vi "asap_stage_calibration.vi"() -> ()   [LabVIEW 2013]
uses:
  <vilib>/Platform/TimedLoop/XDataNode/XDataNode.xnode
  <vilib>/Platform/TimedLoop/XDataNode/nitl_modes.ctl
  <vilib>/Platform/TimedLoop/XDataNode/XDNodeRunTimeDep.lvlib
  <vilib>/Platform/TimedLoop/XDataNode/wakeup.ctl
  <vilib>/Platform/TimedLoop/XDataNode/timing_clust.ctl
  initialization/micron_globals.vi
  <vilib>/Analysis/Matrix/Datatypes/RealMatrix.ctl
  <vilib>/Analysis/Matrix/NI_Matrix.lvlib
  point_selector.ctl
panel:
  in  "Point selector":T1={"Pose mode"=enum."Handle", "Light number"=0} {"Light number" min=0 max=5}
  in  "Pessimize":bool
  in  "Zero Rx":bool
  in  "Home pose offset":dbl[](array[numeric])=[0.0, 0.0, 0.0, 0.0, 0.0, 0.0] format="%#.3f"
  in  "End transform offset":dbl[](array[numeric])=[0.0, 0.0, 0.0, 0.0, 0.0, 0.0] format="%#.3f"
  in  "Update axes":bool
  out "Axis offsets":dbl[](array[numeric])=[0.09384767289236115, -1.0269022597345072, 2.2800407915457908] format="%#.3g"
  in  "LED enable":bool[](array[boolean])=[TRUE, TRUE, TRUE, TRUE, TRUE, TRUE]
  out "Axis scale errors (percent)":sgl[](array[numeric]) format="%#.2f"
  out "End transform string":string
  in  "End transform\ncoordinates":T2(ring)=enum."ASAP"
  in  "Go home":bool
  in  "Clear":bool
  in  "Set home":bool
  out "End transform (stage)":dbl[](array[numeric])=[0.25469575119784055, -16.45995133588347, 3.732397870471535, 0.0, 0.0, 0.0] format="%#.3f"
  in  "Range (degrees)":dbl=40.0 caption="(degrees)"
  in  "Range (mm)":dbl=50.0 caption="(mm)"
  out "Goal pose ASAP string":string
  out "Probe rotation (stage)":T3 format="%#_3f"
  out "Light rotation string":string
  out "Light pose string":string
  out "Probe pose (ASAP)":T3 format="%#_3f"
  out "State orientation string":string
  out "ASAP origin (Base)":dbl[](array[numeric])=[0.0, 0.0, 0.0, 0.0, 0.0, -30.0] format="%#_3p"
  out "Home pose (base)":dbl[](array[numeric])=[0.25469575119784055, -16.45995133588347, 3.732397870471535, 0.0, 0.0, 0.0] format="%#.3f"
  out "Goal pose (stage)":dbl[](array[numeric])=[0.0, 0.0, 0.0, 0.0, 0.0, -30.0] format="%#_3p"
  in  "Go to":bool
  in  "Probe goal pose (ASAP)":dbl[](array[numeric])=[0.0, 0.0, 0.0, 0.0, 0.0, 180.0]
  in  "Update pivot":bool
  out "Off axis":dbl[](array[numeric]) format="%#_3p"
  in  "Pivot point (mm)":dbl[](array[numeric])=[0.09384767289236115, -1.0269022597345072, 2.2800407915457908] format="%#.3g"
  out "Center offsets  (um)":dbl[][](array[numeric]) format="%#_3p"
  in  "Axes":i32[](array[numeric])=[0, 1, 2]
  in  "Find center":bool
  in  "stop":bool
  in  "Find pose":bool
  out "Axis angle errors (radians)":dbl[](array[numeric]) format="%#_3p"
  out "Base orientation (ASAP)":T3 format="%#_3f"
  # "Range limits"
  # "XY"
  # "XZ"
  # "YZ"
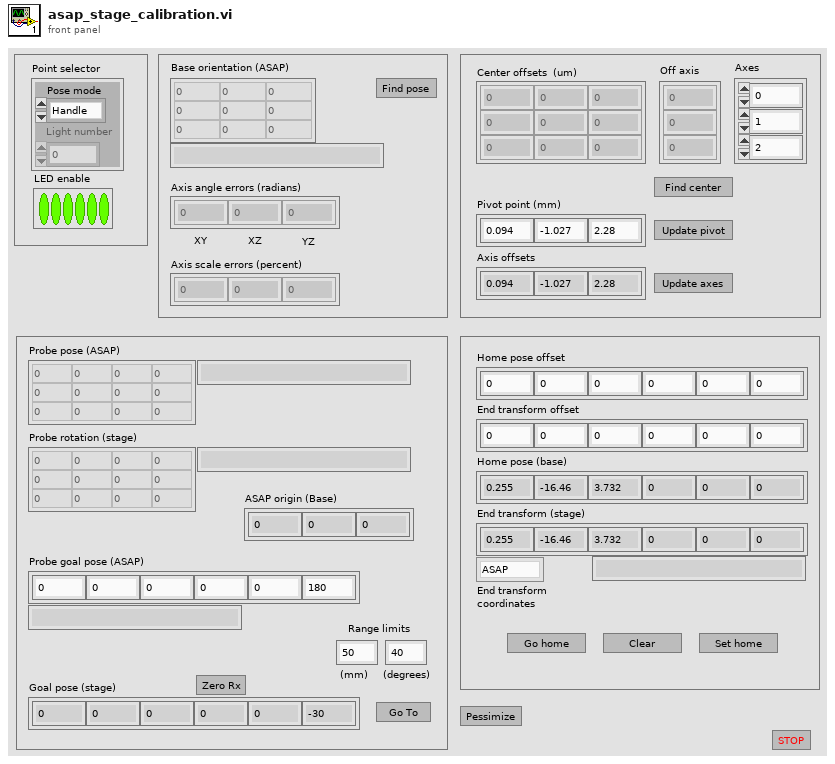
[diagram p1: front panel]
types:
  T1 = typedef "point_selector.ctl" = cluster{"Pose mode":enum16{"Light", "Handle", "Output"}, "Light number":i32}
  T2 = enum16{"Pivot", "Probe", "ASAP", "Sensor 0", "Sensor 1"}
  T3 = typedef "NI_Matrix.lvlib/RealMatrix.ctl" = dbl[][]
  T4 = typedef "ui_override_opts.ctl" = cluster{"Triggering":bool, "Parameters":bool, "Stimulus":bool, "Calibration":bool, "Modes":bool}
  T5 = enum8{"Enabled", "Disabled", "Disabled and Grayed Out"}
  T6 = typedef "XDNodeRunTimeDep.lvlib/timing_clust.ctl" = cluster{"Expected End [f-1]":u64, "Actual End [f-1]":u64, "Finished Late? [f-1]":bool, "Expected End [i-1]":u64, "Actual End [i-1]":u64, "Finished Late? [i-1]":bool, "Expected Start [i]":u64, "Actual Start [i]":u64, "Expected Start [f]":u64, "Actual Start [f]":u64, "Source Name":string, "Structure Name":string, "Period":i64, "Deadline":i64, "Offset":i64, "Start":i64, "Priority":i32, "Timeout":i32, "Mode":T7, "Wakeup Reason":T8, "Error":errorcluster, "Source Type":string, "Secondary Source Type":string, "Global End Time":u64, "Global Start Time":u64, "Frame Duration":u64, "Iteration Duration":u64, "Assigned CPU":i32, "I/O Scan Engine Mode":u32}
  T7 = typedef "XDNodeRunTimeDep.lvlib/nitl_modes.ctl" = enum32{"No Change", "Process missed periods, maintain original phase", "Discard missed periods, maintain original phase", "Process missed periods, ignore original phase", "Discard missed periods, ignore original phase"}
  T8 = typedef "XDNodeRunTimeDep.lvlib/wakeup.ctl" = enum32{"Normal", "Aborted", "Asynchronous wakeup", "Timing source error", "Timed loop error", "Timeout"}
  T9 = typedef "motion_status.ctl" = cluster{"Axis names":string[], "Axis positions":dbl[], "Pose":dbl[], "Timestamp":u32, "Ready":bool, "Stopped":bool}
  T10 = typedef "micron_config.ctl" = cluster{"rt fifo":refnum<k33>, "Analog output task":refnum<k21>, "Analog output task 2":refnum<k21>, "Stimulus AO task":refnum<k21>, "Low-rate AIN task":refnum<k21>, "Pedal out task":refnum<k21>, "Pedal in task":refnum<k21>, "Loop timing source":string, "Relay out task":refnum<k21>, "Send UDP Conn":refnum<k16>, "Recv UDP Conn":refnum<k16>, "Host Addr":dbl, "I2C interface":T11, "trace_start notifier":refnum<notifier>, "trace_done notifier":refnum<notifier>, "ASAP FIFO":refnum<k33>}
  T11 = typedef "i2c_interface.ctl" = cluster{"FPGA VI Reference":T12}
  T12 = typedef "fpga_reference.ctl" = refnum<k20>
  T13 = enum32{"Bad", "Idle", "Run top level", "Running"}
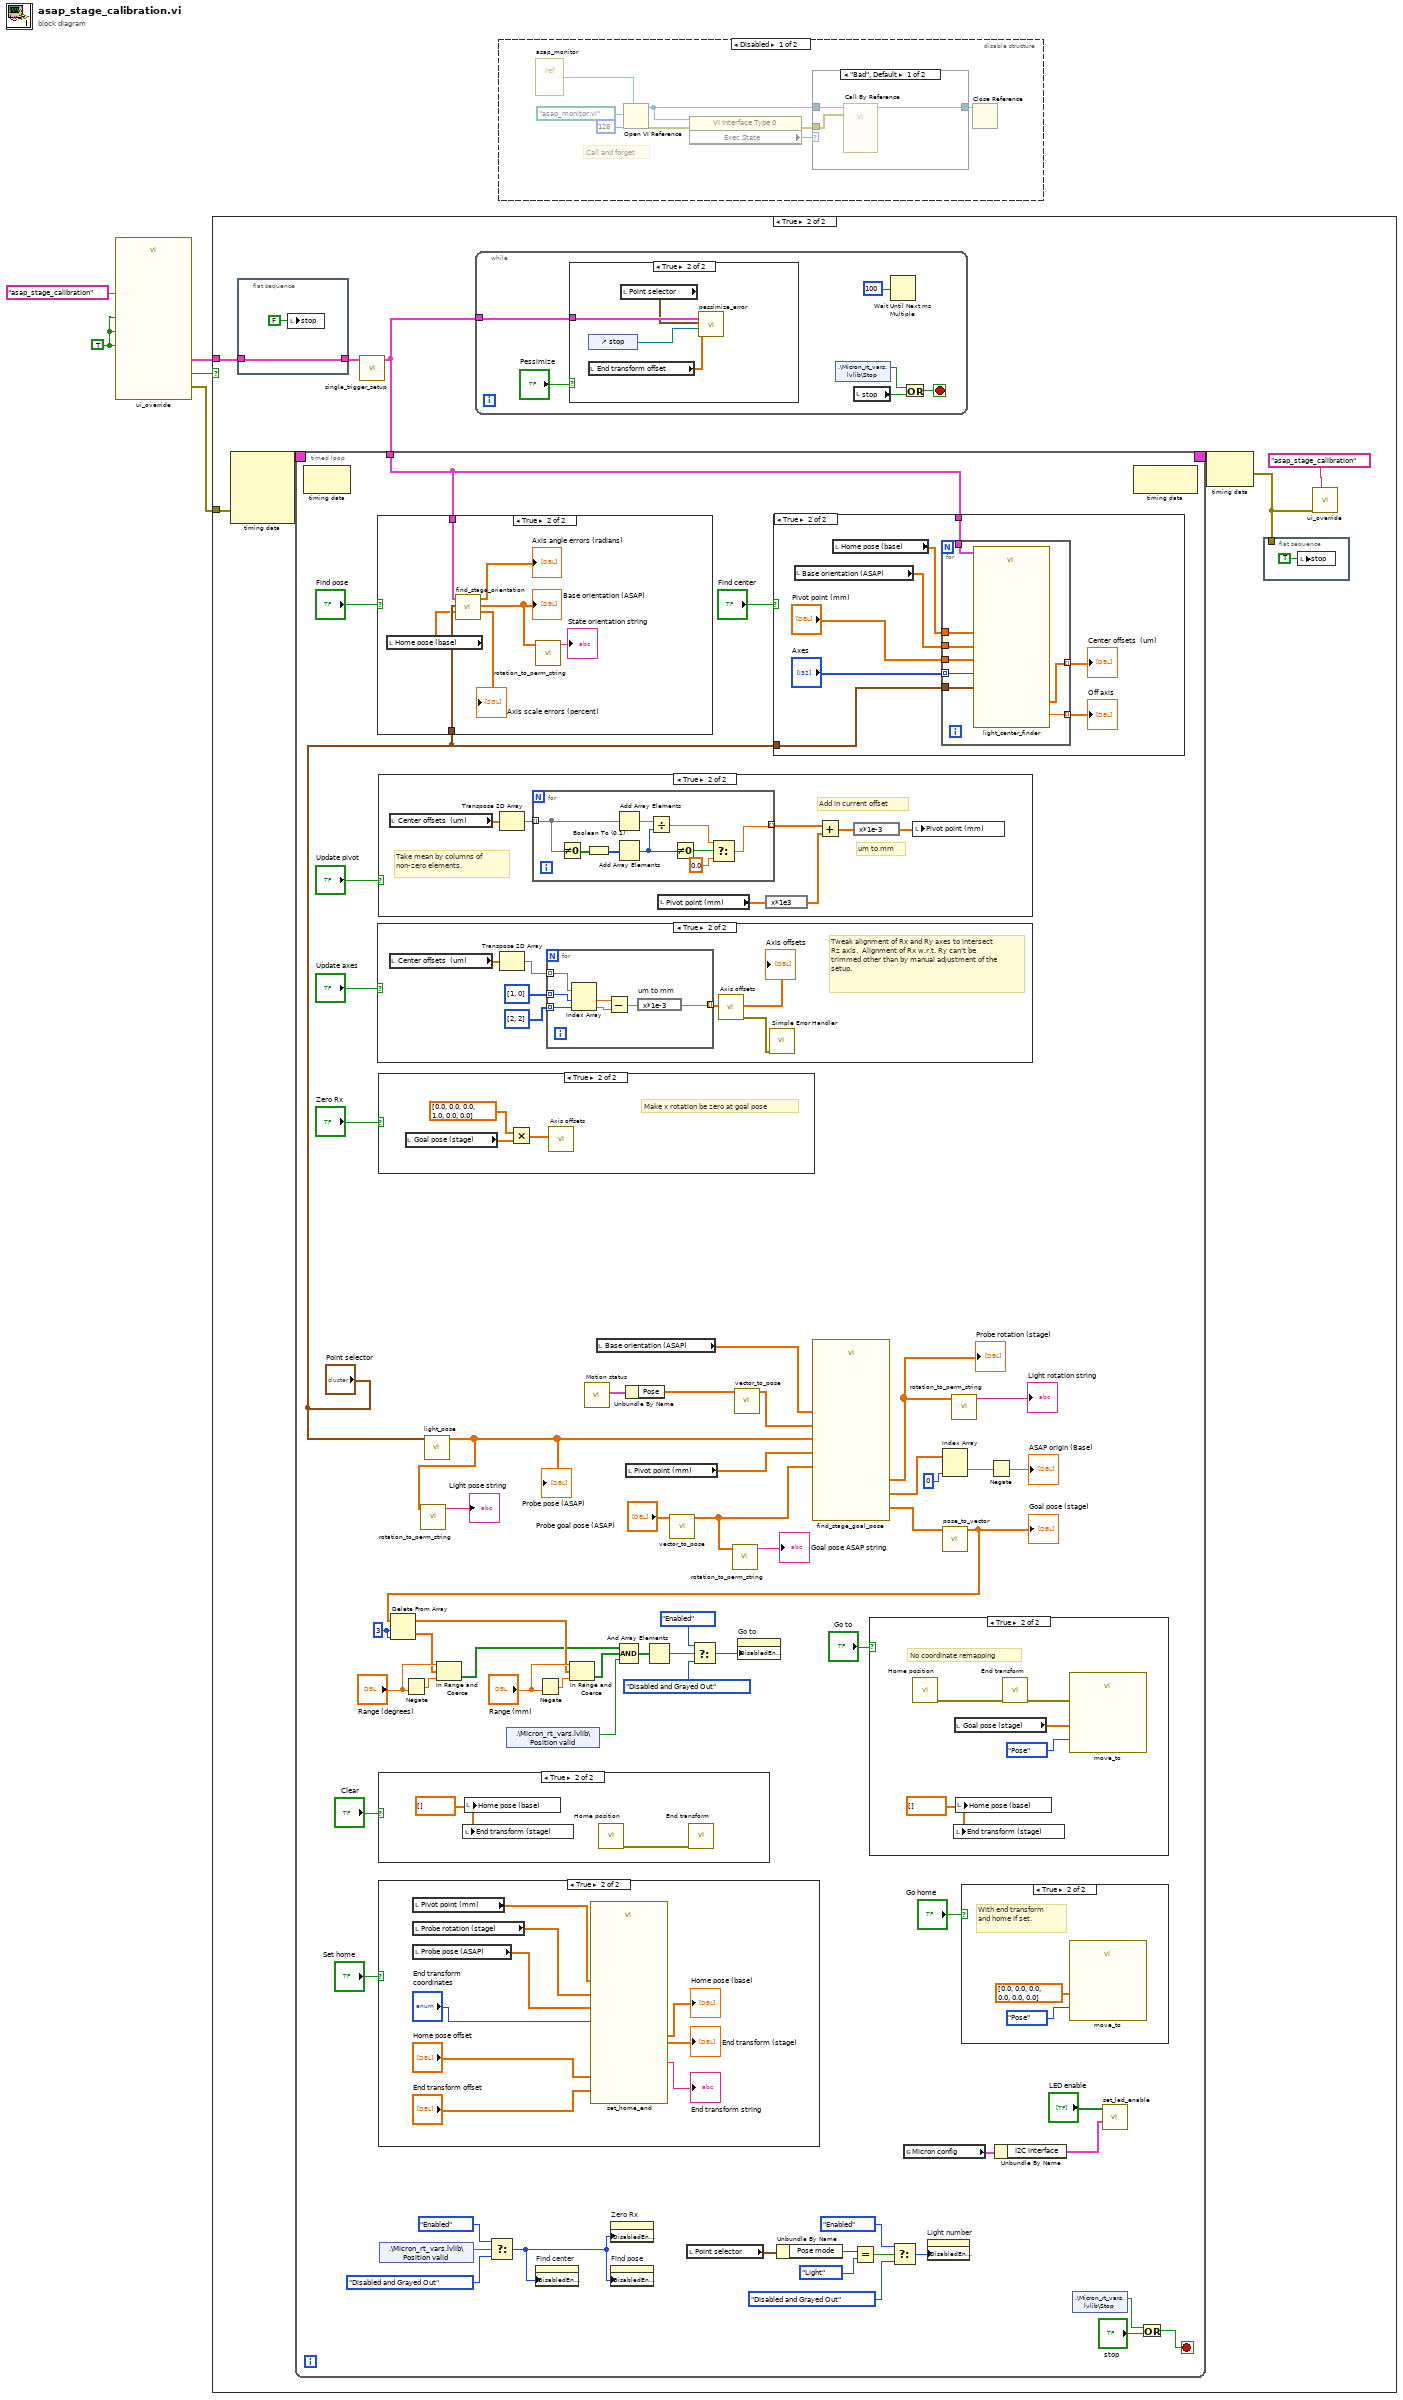
[diagram p0: block diagram]
diagram:
  w3 = TRUE ("Triggering")
  n1 = call "ui_override.vi"("Triggering"=w3, "VI name"="asap_stage_calibration", "Stimulus"=w3, "All or nothing"=w3) -> ("Override"=w2:T4, "Got all"=w5:bool, "error out"=w1:errorcluster)  [unwired: 9 in]
  n2 = case shown="True" w5 {
    tunnel: w1 -> [_ w11]
    tunnel: w2 -> [_ w8]
    frame False {
    }
    frame True {
      n3 = node-c288(w11) -> (w13:T6)  [unwired: 3 in]
      n4 = flat-sequence {
        tunnel: w8 -> [w16]
        tunnel: [w16] -> w9
        frame #0 {
          n5 = local write "stop"(FALSE ("stop")) -> ()
        }
      }
      n6 = call "single_trigger_setup.vi"("Override in"=w9) -> ("Override out"=w7:T4)  [unwired: 10 in]
      n7 = timed-loop {
        timing: w13 -> [_]
        timing-out: [_] -> w12
        tunnel: w7 -> [w83]
        stop <- w84 stop-if-true
        w62 = 3 ("length")
        n8 = node-c288() -> ()  [unwired: 1 in, 1 out]
        n9 = case shown="True" "Find pose" {
          tunnel: w83 -> [_ w161]
          tunnel: "Point selector" -> [_ w159]
          frame False {
          }
          frame True {
            n10 = local read "Home pose (base)"() -> (w158:dbl[])
            n11 = call "find_stage_orientation.vi"("Home pose"=w158, "Point selector"=w159, "Override"=w161) -> ("Axis scale errors (percent)"=→"Axis scale errors (percent)":sgl[], "Stage pose (rotation only)"=w156:T3, "Axis errors (radians)"=→"Axis angle errors (radians)":dbl[])  [unwired: 6 in]
            "Base orientation (ASAP)" <- w156
            n12 = call "rotation_to_perm_string.vi"("Rotation matrix (T)"=w156) -> ("Axis permutation and residue"=→"State orientation string":string)  [unwired: 10 in]
          }
        }
        n13 = case shown="True" "Update axes" {
          frame False {
          }
          frame True {
            # "Tweak alignment of Rx and Ry axes to intersect Rz axis.  Alignment of Rx w.r.t. Ry can't be trimmed other than by manual adjustment of the setup."
            n14 = local read "Center offsets  (um)"() -> (w96:dbl[][])
            n15 = Transpose 2D Array(2D array=w96) -> (transposed array=w95:dbl[][])
            n16 = for {
              tunnel: w95 -> [w102] mode=indexing
              tunnel: i32[] [1, 0] -> [w104] mode=indexing
              tunnel: i32[] [2, 2] -> [w103] mode=indexing
              tunnel: [w98] -> w92 mode=indexing
              n17 = Index Array(array=w102, index #1=w104, index #2=w103) -> (element #1=w101:dbl, element #2=w100:dbl)
              n18 = Subtract(x=w101, y=w100) -> (x-y=w99:dbl)
              n19 = expression code="x*1e-3" "um to mm"(w99) -> (w98:dbl)
            }
            n20 = call "Axis offsets.vi"("Axis offsets increment"=w92) -> ("error out"=w91:errorcluster, "Axis offsets"=→"Axis offsets":dbl[])  [unwired: 9 in]
            n21 = call <vilib>:"Simple Error Handler.vi"("error in (no error)"=w91) -> ()  [unwired: 4 in, 5 out]
          }
        }
        n22 = case shown="True" "Update pivot" {
          frame False {
          }
          frame True {
            # "Add in current offset"
            # "um to mm"
            # "Take mean by columns of non-zero elements."
            n23 = local read "Center offsets  (um)"() -> (w129:dbl[][])
            n24 = Transpose 2D Array(2D array=w129) -> (transposed array=w128:dbl[][])
            n25 = for {
              tunnel: w128 -> [w136] mode=indexing
              tunnel: [w131] -> w126 mode=indexing
              n26 = Not Equal To 0?(x=w136) -> (x != 0?=w138:bool[])
              n27 = Boolean To (0,1)(Boolean=w138) -> (0, 1=w137:i16[])
              n28 = Add Array Elements(numeric array=w136) -> (sum=w135:dbl)
              n29 = Add Array Elements(numeric array=w137) -> (sum=w134:i16)
              n30 = Divide(x=w135, y=w134) -> (x/y=w132:dbl)
              n31 = Not Equal To 0?(x=w134) -> (x != 0?=w133:bool)
              n32 = Select(t=w132, s=w133, f=0.0) -> (s? t:f=w131:dbl)
            }
            n33 = local read "Pivot point (mm)"() -> (w124:dbl[])
            n34 = expression code="x*1e3"(w124) -> (w123:dbl[])
            n35 = Add(x=w126, y=w123) -> (x+y=w125:dbl[])
            n36 = expression code="x*1e-3"(w125) -> (w127:dbl[])
            n37 = local write "Pivot point (mm)"(w127) -> ()
          }
        }
        n38 = case shown="True" "Zero Rx" {
          frame False {
          }
          frame True {
            # "Make x rotation be zero at goal pose"
            n39 = local read "Goal pose (stage)"() -> (w90:dbl[])
            n40 = Multiply(x=dbl[] [0.0, 0.0, 0.0, 1.0, 0.0, 0.0] ("Goal pose (stage)"), y=w90) -> (x*y=w88:dbl[])
            n41 = call "Axis offsets.vi"("Axis offsets increment"=w88) -> ()  [unwired: 9 in, 2 out]
          }
        }
        n42 = case shown="True" "Clear" {
          frame False {
          }
          frame True {
            w107 = dbl[] [] ("Home position")
            n43 = local write "End transform (stage)"(w107) -> ()
            n44 = local write "Home pose (base)"(w107) -> ()
            n45 = call "Home position.vi"() -> ("error out"=w108:errorcluster)  [unwired: 11 in]
            n46 = call "End transform.vi"("error in"=w108) -> ()  [unwired: 10 in, 1 out]
          }
        }
        n47 = case shown="True" "Set home" {
          frame False {
          }
          frame True {
            n48 = local read "Pivot point (mm)"() -> (w116:dbl[])
            n49 = local read "Probe rotation (stage)"() -> (w115:T3)
            n50 = local read "Probe pose (ASAP)"() -> (w112:T3)
            n51 = call "set_home_end.vi"("End transform offset"="End transform offset", "End transform coordinates"="End transform\ncoordinates", "Home pose offset"="Home pose offset", "Probe pose (ASAP)"=w112, "Probe rotation (stage)"=w115, "Pivot point (mm)"=w116) -> ("End transform string"=→"End transform string":string, "End transform"=→"End transform (stage)":dbl[], "Home pose"=→"Home pose (base)":dbl[])  [unwired: 3 in]
          }
        }
        n52 = shared-variable ".\\Micron_rt_vars.lvlib\\Position valid"() -> (w40:bool)  [unwired: 1 in, 1 out]
        n53 = Negate(x="Range (degrees)") -> (-x=w59:dbl)
        n54 = call "light_pose.vi"("Point selector"="Point selector") -> ("Light pose (ASAP coordinates)"=w66:T3)  [unwired: 10 in]
        "Probe pose (ASAP)" <- w66
        n55 = call "rotation_to_perm_string.vi"("Rotation matrix (T)"=w66) -> ("Axis permutation and residue"=→"Light pose string":string)  [unwired: 10 in]
        n56 = Select(t=T5."Enabled" ("Disabled"), s=w40, f=T5."Disabled and Grayed Out" ("Disabled")) -> (s? t:f=w35:T5)
        n57 = shared-variable ".\\Micron_rt_vars.lvlib\\Position valid"() -> (w37:bool)  [unwired: 1 in, 1 out]
        n58 = property on="Find center" class="Bool"("DisabledEnum"=w35) -> ()  [unwired: 2 in, 2 out]
        n59 = Negate(x="Range (mm)") -> (-x=w61:dbl)
        n60 = call "Motion status.vi"() -> ("Motion status"=w79:T9)  [unwired: 6 in, 5 out]
        n61 = local read "Base orientation (ASAP)"() -> (w70:T3)
        n62 = property on="Zero Rx" class="Bool"("DisabledEnum"=w35) -> ()  [unwired: 2 in, 2 out]
        n63 = property on="Find pose" class="Bool"("DisabledEnum"=w35) -> ()  [unwired: 2 in, 2 out]
        n64 = Unbundle By Name(w79) -> ("Pose"=w76:dbl[])
        n65 = local read "Pivot point (mm)"() -> (w77:dbl[])
        n66 = call "vector_to_pose.vi"("Pose vector"="Probe goal pose (ASAP)") -> ("Pose"=w65:T3)  [unwired: 10 in]
        n67 = local read "Point selector"() -> (w29:T1)
        n68 = call "rotation_to_perm_string.vi"("Rotation matrix (T)"=w65) -> ("Axis permutation and residue"=→"Goal pose ASAP string":string)  [unwired: 10 in]
        n69 = call "vector_to_pose.vi"("Pose vector"=w76) -> ("Pose"=w71:T3)  [unwired: 10 in]
        n70 = case shown="True" "Find center" {
          tunnel: w83 -> [_ w146]
          tunnel: "Point selector" -> [_ w145]
          frame False {
          }
          frame True {
            n71 = local read "Base orientation (ASAP)"() -> (w142:T3)
            n72 = local read "Home pose (base)"() -> (w140:dbl[])
            n73 = for {
              tunnel: w146 -> [w154]
              tunnel: w145 -> [w153]
              tunnel: "Axes" -> [w152] mode=indexing
              tunnel: [w151] -> w143 mode=indexing
              tunnel: [w150] -> w141 mode=indexing
              tunnel: w142 -> [w149]
              tunnel: "Pivot point (mm)" -> [w148]
              tunnel: w140 -> [w147]
              n74 = call "light_center_finder.vi"("Home pose"=w147, "Stage orientation"=w149, "Pivot point"=w148, "Point selector"=w153, "Axis"=w152, "Override"=w154) -> ("Light offset (stage coords)"=w151:dbl[], "Off axis"=w150:dbl)  [unwired: 3 in, 1 out]
            }
            "Center offsets  (um)" <- w143
            "Off axis" <- w141
          }
        }
        n75 = Unbundle By Name(w29) -> ("Pose mode"=w28:enum16{"Light", "Handle", "Output"})
        n76 = call "find_stage_goal_pose.vi"("Pivot point (mm)"=w77, "G^A: Goal (ASAP)"=w65, "L^A: Light pose (ASAP)"=w66, "E^B: current stage pose (base)"=w71, "O^A: base Orientation (ASAP)"=w70) -> ("E'^B: goal pose (Base)"=w72:T3, "t^O: translation ASAP -> base"=w74:T3, "L^P: rotation of lights (Pivot)"=w68:T3)  [unwired: 4 in]
        "Probe rotation (stage)" <- w68
        n77 = Equal?(x=w28, y=enum16{"Light", "Handle", "Output"}."Light" ("Pose mode")) -> (x = y?=w32:bool)
        n78 = case shown="True" "Go to" {
          frame False {
          }
          frame True {
            w118 = dbl[] [] ("Home position")
            # "No coordinate remapping"
            n79 = call "Home position.vi"() -> ("error out"=w120:errorcluster)  [unwired: 11 in]
            n80 = local write "End transform (stage)"(w118) -> ()
            n81 = local read "Goal pose (stage)"() -> (w121:dbl[])
            n82 = local write "Home pose (base)"(w118) -> ()
            n83 = call "End transform.vi"("error in"=w120) -> ("error out"=w119:errorcluster)  [unwired: 10 in]
            n84 = call "move_to.vi"("Error in"=w119, "Axis positions"=w121, "Mode"=enum16{"Absolute axis", "Relative axis", "Pose"}."Pose") -> ()  [unwired: 8 in, 1 out]
          }
        }
        n85 = Select(t=T5."Enabled" ("Disabled"), s=w32, f=T5."Disabled and Grayed Out" ("Disabled")) -> (s? t:f=w27:T5)
        n86 = global read "micron_globals.vi" "Micron config"() -> (w43:T10)
        n87 = property on="Light number" class="DigNum (strict)"("DisabledEnum"=w27) -> ()  [unwired: 2 in, 2 out]
        n88 = Index Array(array=w74, index (col)=0 ("disabled index (col)")) -> (element=w46:dbl[])  [unwired: 1 in]
        n89 = call "pose_to_vector.vi"("Pose"=w72) -> ("Pose vector"=w63:dbl[])  [unwired: 10 in]
        "Goal pose (stage)" <- w63
        n90 = Delete From Array(array=w63, length=w62, index=w62) -> (deleted portion=w56:dbl[], array with subset deleted=w57:dbl[])
        n91 = In Range and Coerce(upper limit="Range (degrees)", x=w56, lower limit=w59) -> (In Range?=w55:bool[])  [unwired: 1 out]
        n92 = In Range and Coerce(upper limit="Range (mm)", x=w57, lower limit=w61) -> (In Range?=w54:bool[])  [unwired: 1 out]
        n93 = Compound Arithmetic op=AND(w55, w54, w37) -> (w53:bool[])
        n94 = And Array Elements(Boolean array=w53) -> (logical AND=w50:bool)
        n95 = Select(t=T5."Enabled" ("Disabled"), s=w50, f=T5."Disabled and Grayed Out" ("Disabled")) -> (s? t:f=w49:T5)
        n96 = property on="Go to" class="Bool"("DisabledEnum"=w49) -> ()  [unwired: 2 in, 2 out]
        n97 = call "rotation_to_perm_string.vi"("Rotation matrix (T)"=w68) -> ("Axis permutation and residue"=→"Light rotation string":string)  [unwired: 10 in]
        n98 = case shown="True" "Go home" {
          frame False {
          }
          frame True {
            # "With end transform and home if set."
            n99 = call "move_to.vi"("Axis positions"=dbl[] [0.0, 0.0, 0.0, 0.0, 0.0, 0.0], "Mode"=enum16{"Absolute axis", "Relative axis", "Pose"}."Pose") -> ()  [unwired: 9 in, 1 out]
          }
        }
        n100 = Negate(x=w46) -> (-x=→"ASAP origin (Base)":dbl[])
        n101 = Unbundle By Name(w43) -> ("I2C interface"=w42:T11)
        n102 = shared-variable ".\\Micron_rt_vars.lvlib\\Stop"() -> (w86:bool)  [unwired: 1 in, 1 out]
        n103 = call "set_led_enable.vi"("I2C interface"=w42, "LED enables"="LED enable") -> ()  [unwired: 9 in, 1 out]
        n104 = node-c288() -> ()  [unwired: 1 in, 1 out]
        n105 = Or(x=w86, y="stop") -> (x .or. y?=w84:bool)
      }
      n106 = while {
        tunnel: w7 -> [w21]
        stop <- w18 stop-if-true
        n107 = case shown="True" "Pessimize" {
          tunnel: w21 -> [_ w26]
          frame False {
          }
          frame True {
            n108 = control-ref of="stop"() -> (w24:refnum<vi>)
            n109 = local read "End transform offset"() -> (w23:dbl[])
            n110 = local read "Point selector"() -> (w25:T1)
            n111 = call "pessimize_error.vi"("End transform offset"=w23, "stop"=w24, "Point selector"=w25, "Override in"=w26) -> ()  [unwired: 8 in]
          }
        }
        n112 = shared-variable ".\\Micron_rt_vars.lvlib\\Stop"() -> (w20:bool)  [unwired: 1 in, 1 out]
        n113 = local read "stop"() -> (w19:bool)
        n114 = Wait Until Next ms Multiple(millisecond multiple=u32 100) -> ()  [unwired: 1 out]
        n115 = Or(x=w20, y=w19) -> (x .or. y?=w18:bool)
      }
      n116 = node-c288(w12) -> (w6:errorcluster)
      n117 = flat-sequence {
        tunnel: w6 -> [_]
        frame #0 {
          n118 = local write "stop"(TRUE ("stop")) -> ()
        }
      }
      n119 = call "ui_override.vi"("VI name"="asap_stage_calibration", "error in"=w6) -> ()  [unwired: 11 in, 3 out]
    }
  }
  n120 = disable-structure shown="Disabled" {
    frame Disabled {
      # "Call and forget"
      n121 = vi-ref "asap_monitor.vi"() -> (w174:refnum<vi>)
      n122 = Open VI Reference(type specifier VI Refnum (for type only)=w174, vi path=path "asap_monitor.vi", options=128) -> (vi reference=w173:refnum<vi>, error out=w172:errorcluster)  [unwired: 3 in]
      n123 = property class="VI Interface Type 0"(reference=w173, error in=w172) -> (error out=w169:errorcluster, "Exec.State"=w170:T13)  [unwired: 1 out]
      n124 = case shown="\"Bad\", Default" w170 {
        tunnel: w173 -> [w179 w180]
        tunnel: [w178 w180] -> w171
        tunnel: w169 -> [w177 _]
        frame "Bad", Default {
          n125 = call-by-ref "Call By Reference"(reference=w179, error in=w177) -> (reference out=w178:refnum<vi>)  [unwired: 12 in, 1 out]
        }
        frame "Run top level", "Running" {
        }
      }
      n126 = Close Reference(reference=w171) -> ()  [unwired: 1 in, 1 out]
    }
    frame Enabled {
    }
  }
